vi "SaveSystemConfigurationUI.vi"(8 "error in (no error)":errorcluster, 11 "TestSetup in":refnum<class "TestSetup.lvclass">) -> (0 "error out":errorcluster, 3 "TestSetup out":refnum<class "TestSetup.lvclass">)   [LabVIEW 2019, in "TestSetup.lvlib" / "TestSetup.lvclass"]
uses:
  TestSetup.lvclass
  C:/Program Files (x86)/National Instruments/LabVIEW 2019/vi.lib/NI/Event Source Actor/Event Source/Event Source/Event Source.lvclass
  TestSetup.lvclass/TestSetup.ctl
  SystemSetup/SystemSetup/SystemConfiguration.lvclass
  C:/Program Files (x86)/National Instruments/LabVIEW 2019/vi.lib/NI/Event Source Actor/Event Source/Event/Event.lvclass
  <vilib>/NI/Event Source Actor/Event Source/Event/Event.lvclass/Event.ctl
  <vilib>/Utility/file.llb/Write Delimited Spreadsheet (string).vi
  SystemSetup/SystemSetup/SystemSetup.lvclass
  <vilib>/NI/Event Source Actor/Event Source/Event Source/Event Source.lvclass
  <vilib>/NI/Event Source Actor/Event Source/Event/Event.lvclass
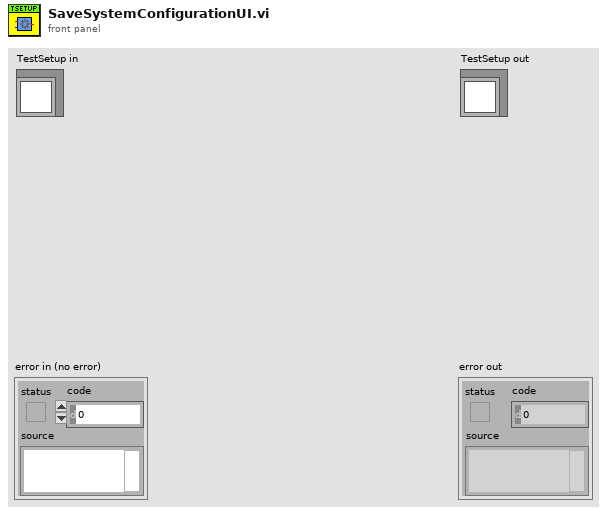
[diagram p1: front panel]
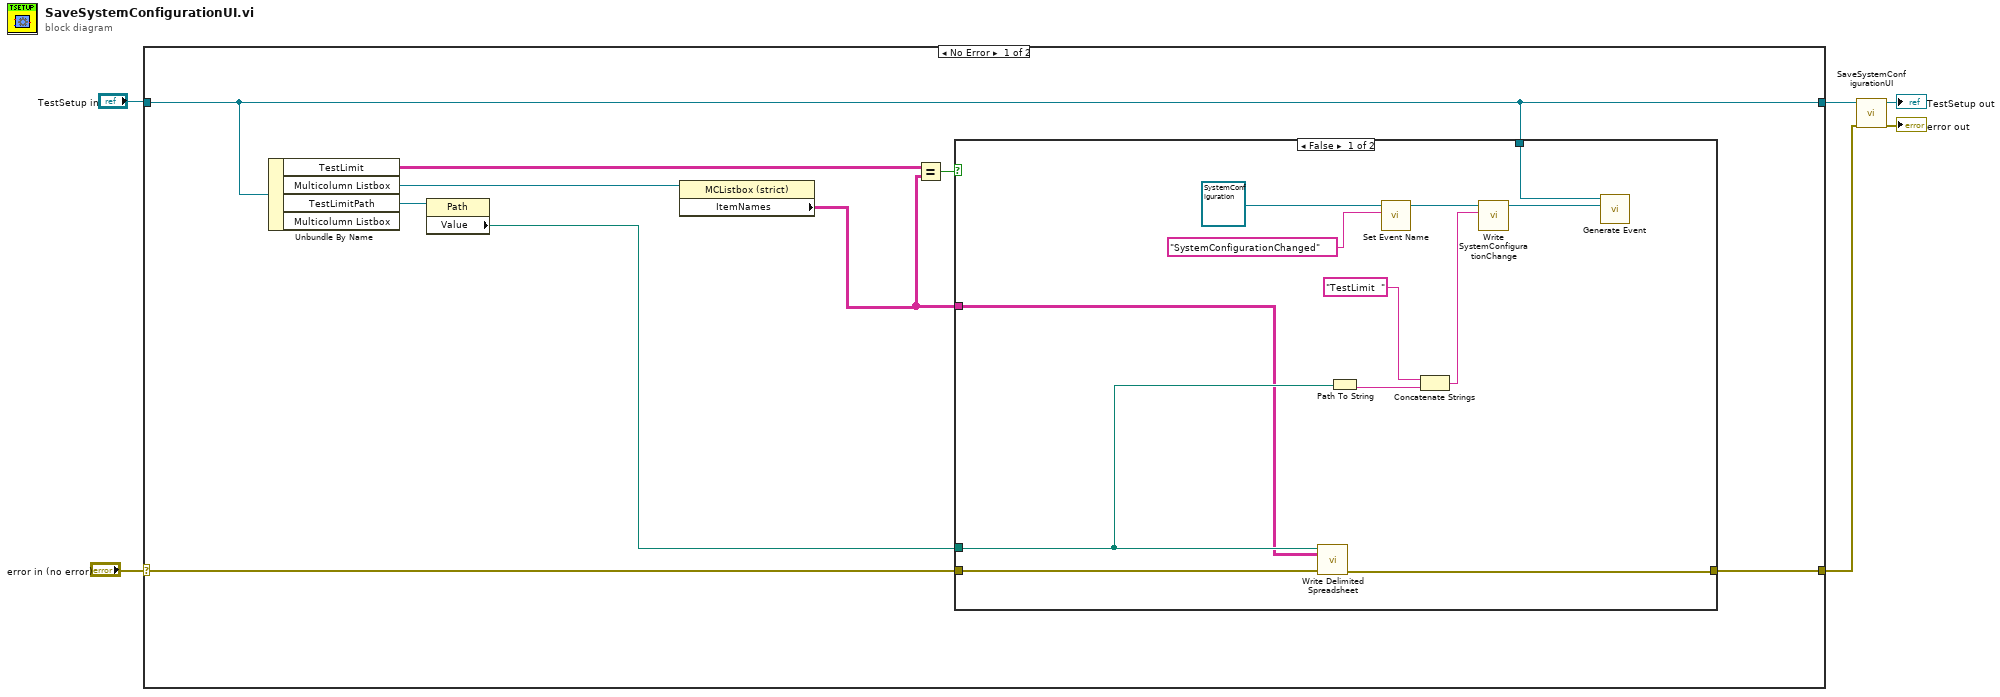
[diagram p0: block diagram]
diagram:
  n1 = case shown="No Error" "error in (no error)" {
    selector: "error in (no error)" -> [w14 w30]
    tunnel: [w13 w30] -> w1
    tunnel: [w10 w29] -> w2
    tunnel: "TestSetup in" -> [w10 w29]
    frame No Error {
      n2 = Unbundle By Name(w10) -> ("TestLimit"=w12:string[][], "Multicolumn Listbox"=w15:refnum<vi>, "TestLimitPath"=w9:refnum<vi>)  [unwired: 1 out]
      n3 = property class="Path"(reference=w9) -> ("Value"=w8:path)  [unwired: 1 in, 2 out]
      n4 = property class="MCListbox (strict)"(reference=w15) -> ("ItemNames"=w7:string[][])  [unwired: 1 in, 2 out]
      n5 = Equal?(x=w12, y=w7) -> (x = y?=w11:bool)
      n6 = case shown="False" w11 {
        tunnel: w14 -> [w25 w28]
        tunnel: [w24 w28] -> w13
        tunnel: w8 -> [w27 _]
        tunnel: w7 -> [w26 _]
        tunnel: w10 -> [w19 _]
        frame False {
          n7 = call-poly <vilib>:"Write Delimited Spreadsheet.vi"("file path (dialog if empty)"=w27, "2D data"=w26, "error in (no error)"=w25) -> ("error out"=w24:errorcluster)  [unwired: 11 in, 1 out]
          n8 = Path To String(path=w27) -> (string=w17:string)
          n9 = call <vilib>:"Set Event Name.vi"("Name (Generic)"="SystemConfigurationChanged", "Event In"=refnum<class "SystemConfiguration.lvclass"> refnum ("SystemSetup.lvlib:SystemConfiguration.lvclass")) -> ("Event Out"=w21:refnum<class "SystemConfiguration.lvclass">)  [unwired: 9 in]
          n10 = Concatenate Strings("TestLimit  " ("SystemConfigurationChange"), w17) -> (w16:string)
          n11 = call-dynamic "Write SystemConfigurationChange.vi"("SystemConfigurationChange"=w16, "SystemConfiguration in"=w21) -> ("SystemConfiguration out"=w20:refnum<class "SystemConfiguration.lvclass">)  [unwired: 8 in, 1 out]
          n12 = call <vilib>:"Generate Event.vi"("Event"=w20, "Event Source In"=w19) -> ()  [unwired: 8 in, 2 out]
        }
        frame True {
        }
      }
    }
    frame Error {
    }
  }
  n13 = call-parent "SaveSystemConfigurationUI.vi"("error in (no error)"=w1, "SystemSetup in"=w2) -> ("error out"=→"error out":errorcluster, "SystemSetup out"=→"TestSetup out":refnum<class "TestSetup.lvclass">)  [unwired: 8 in]
